vi "Field Setup.vi"(6 "path to png file":path=path "C:/Users/a0272913/Desktop/AppRawJSON/drawing.png", 10 "JSONCluster":T2, 11 "Zones In":T1[](array[typedef])) -> (2 "Field":picture, 3 "Zones Out":T1[](array[typedef]))   [LabVIEW 2015]
uses:
  Typedef/JSONCluster.ctl
  Typedef/Zone Data.ctl
panel:
  in  "Open Button":bool
  in  "Save Button":bool
  in  "Zones":i32(listbox)
  in  "Close":bool
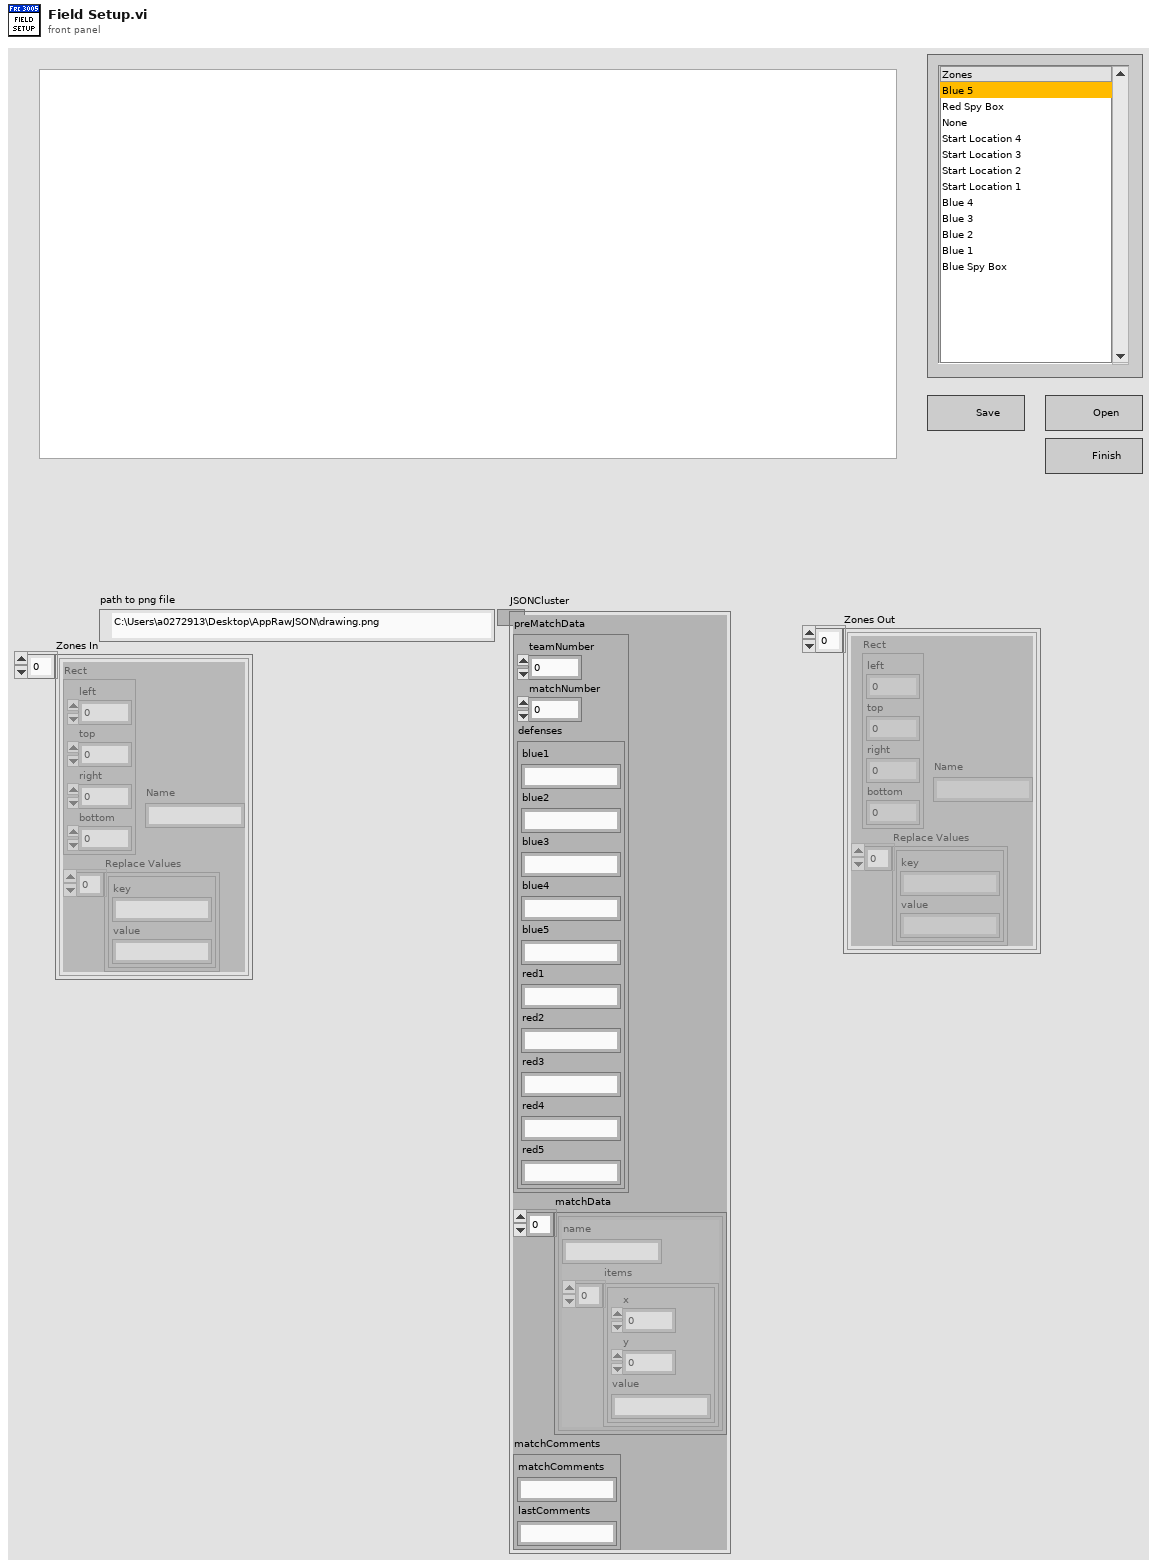
[diagram p1: front panel]
types:
  T1 = typedef "Zone Data.ctl" = cluster{"Rect":cluster{"left":i16, "top":i16, "right":i16, "bottom":i16}, "Replace Values":cluster{"key":string, "value":string}[], "Name":string}
  T2 = typedef "JSONCluster.ctl" = cluster{"preMatchData":cluster{"teamNumber":i32, "matchNumber":i32, "defenses":cluster{"blue1":string, "blue2":string, "blue3":string, "blue4":string, "blue5":string, "red1":string, "red2":string, "red3":string, "red4":string, "red5":string}}, "matchData":cluster{"name":string, "items":cluster{"x":i32, "y":i32, "value":string}[]}[], "matchComments":cluster{"matchComments":string, "lastComments":string}}
  T3 = cluster{"Field":picture, "Zone Active?":bool, "StoredField":picture, "Active Zone":cluster{"TLx":i16, "TLy":i16, "BRx":i16, "BRy":i16}, "Zones":T1[]}
  T4 = typedef "LVBoundsTypeDef.ctl" = cluster{"Width":u32, "Height":u32}
  T5 = typedef "imagedata.ctl" = cluster{"image type":i32, "image depth":i32, "image":u8[], "mask":u8[], "colors":u32[], "Rectangle":cluster{"left":i16, "top":i16, "right":i16, "bottom":i16}}
  T6 = cluster{"name":string, "items":cluster{"x":i32, "y":i32, "value":string}[]}[]
  T7 = typedef "LVMouseTypeDef.ctl" = cluster{"Mouse Position":cluster{"X":i32, "Y":i32}, "Mouse Modifiers":cluster{"Button Down":bool, "Shift Mod":bool, "Menu Mod":bool, "Option Mod":bool}}
  T8 = cluster{"TLx":i16, "TLy":i16, "BRx":i16, "BRy":i16}
  T9 = cluster{"left":i16, "top":i16, "right":i16, "bottom":i16}
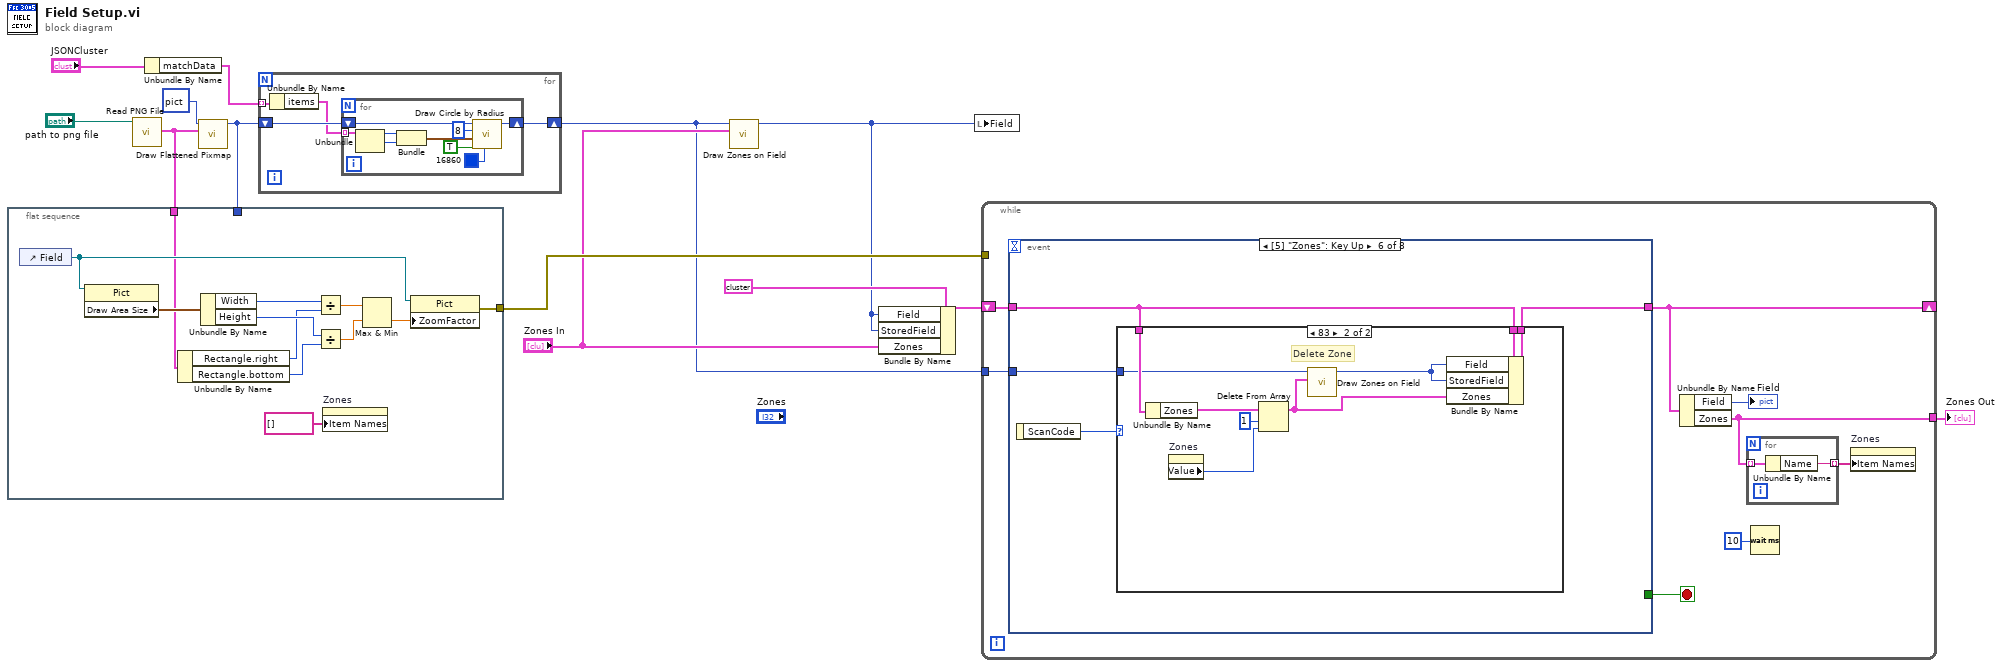
[diagram p0: block diagram]
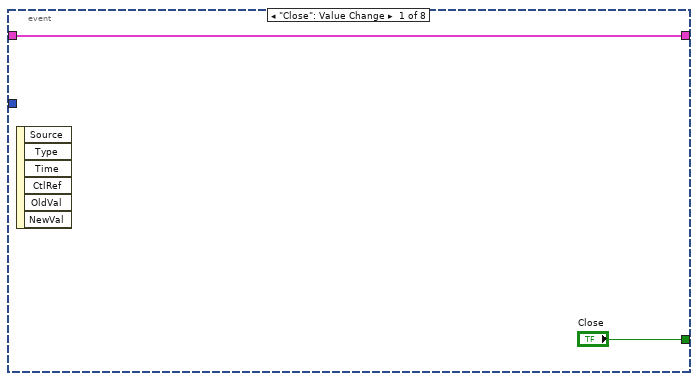
[diagram p2: hidden frame]
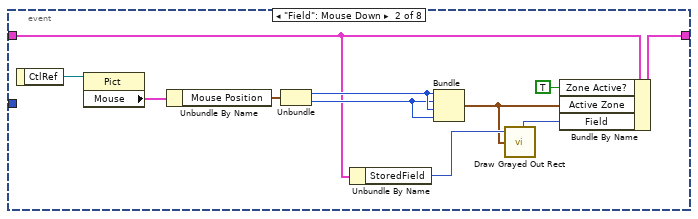
[diagram p3: hidden frame]
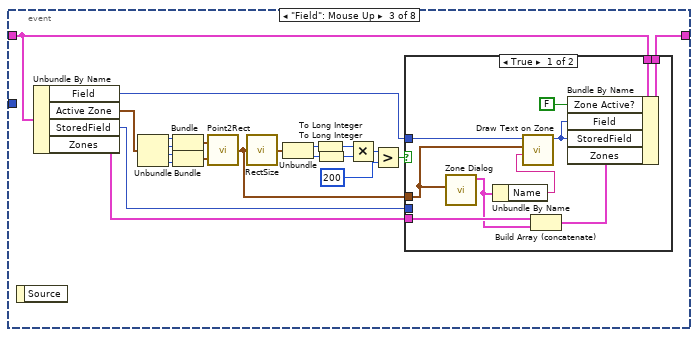
[diagram p4: hidden frame]
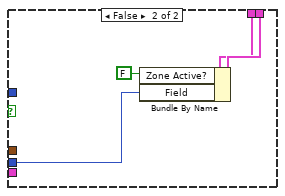
[diagram p5: hidden frame]
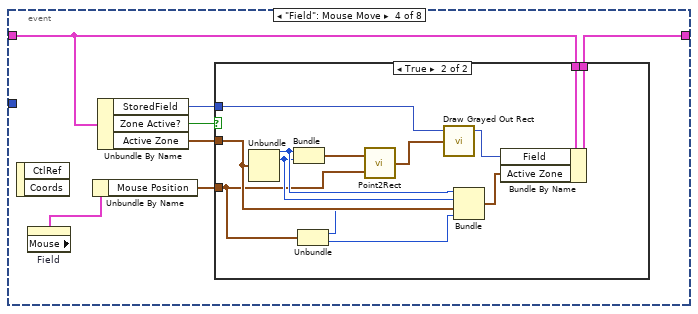
[diagram p6: hidden frame]
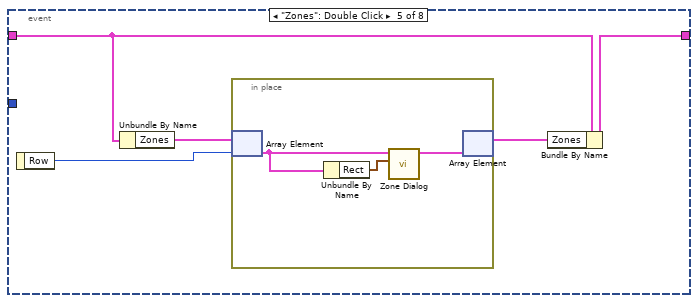
[diagram p8: hidden frame]
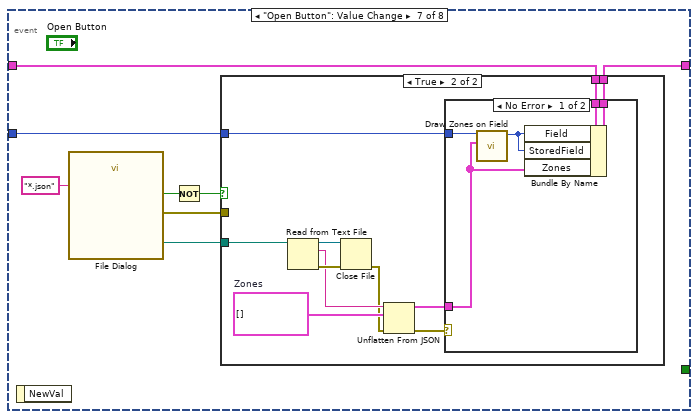
[diagram p10: hidden frame]
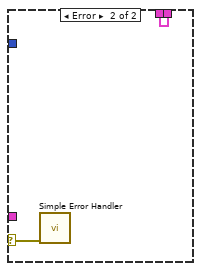
[diagram p12: hidden frame]
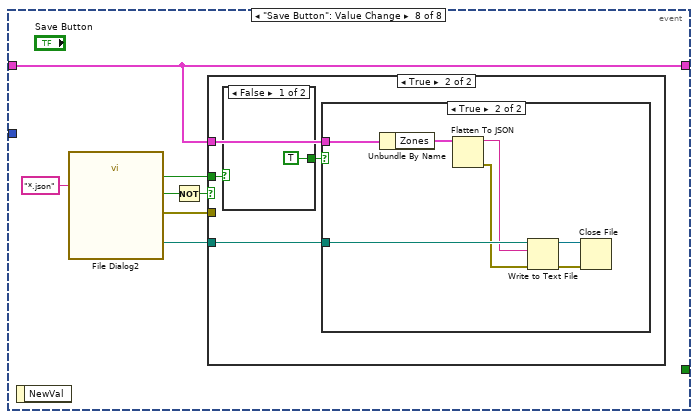
[diagram p13: hidden frame]
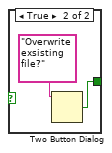
[diagram p15: hidden frame]
diagram:
  n1 = flat-sequence {
    tunnel: w12 -> [w16]
    tunnel: [w15] -> w7
    tunnel: w9 -> [_]
    frame #0 {
      n2 = control-ref of="Field"() -> (w17:refnum<vi>)
      n3 = property class="Pict"(reference=w17) -> ("Draw Area Size"=w22:T4)  [unwired: 1 in, 2 out]
      n4 = Unbundle By Name(w16) -> ("Rectangle.right"=w19:i16, "Rectangle.bottom"=w18:i16)
      n5 = Unbundle By Name(w22) -> ("Width"=w21:u32, "Height"=w20:u32)
      n6 = Divide(x=w21, y=w19) -> (x/y=w23:dbl)
      n7 = Divide(x=w20, y=w18) -> (x/y=w24:dbl)
      n8 = property on="Zones" class="LstBox (strict)"("Item Names"=string[] []) -> ()  [unwired: 2 in, 2 out]
      n9 = Max & Min(x=w23, y=w24) -> (min(x,y)=w25:dbl)  [unwired: 1 out]
      n10 = property class="Pict"(reference=w17, "ZoomFactor"=w25) -> (error out=w15:errorcluster)  [unwired: 1 in, 1 out]
    }
  }
  n11 = call <vilib>:"Read PNG File.vi"("path to PNG file"="path to png file") -> ("image data"=w12:T5)  [unwired: 8 in, 2 out]
  n12 = Unbundle By Name("JSONCluster") -> ("matchData"=w11:T6)
  n13 = call <vilib>:"Draw Flattened Pixmap.vi"("image data"=w12, "picture"=picture data[5B]) -> ("new picture"=w9:picture)  [unwired: 7 in]
  n14 = for {
    shift-right: [w28] -> w1
    shift-left: w9 -> [w29]
    tunnel: w11 -> [w27] mode=indexing
    n15 = Unbundle By Name(w27) -> ("items"=w26:cluster{"x":i32, "y":i32, "value":string}[])
    n16 = for {
      shift-right: [w37] -> w28
      shift-left: w29 -> [w38]
      tunnel: w26 -> [w33] mode=indexing
      n17 = Unbundle(w33) -> ("x"=w32:i32, "y"=w31:i32)  [unwired: 1 out]
      n18 = Bundle("x"=w32, "y"=w31) -> (w30:cluster{"x":i32, "y":i32})  [unwired: 1 in]
      n19 = call <vilib>:"Draw Circle by Radius.vi"("color(black)"=u32 16860, "fill?(F)"=TRUE, "pixel center"=w30, "radius"=i16 8, "picture"=w38) -> ("new picture"=w37:picture)  [unwired: 6 in]
    }
  }
  n20 = call "Draw Zones on Field.vi"("Zones In"="Zones In", "new picture in"=w1) -> ("new picture out"=w3:picture)  [unwired: 9 in]
  n21 = Bundle By Name(cluster=T3 {"Field"=bytes[0], "Zone Active?"=FALSE, "StoredField"=bytes[0], "Active Zone"={"TLx"=0, "TLy"=0, "BRx"=0, "BRy"=0}, "Zones"=[]}, "Field"=w3, "StoredField"=w3, "Zones"="Zones In") -> (w5:T3)
  n22 = local write "Field"(w3) -> ()
  n23 = while {
    tunnel: w7 -> [_]
    shift-right: [w45] -> _
    shift-left: w5 -> [w46]
    tunnel: [w40] -> w4
    tunnel: w1 -> [w39]
    stop <- w43 stop-if-true
    n24 = event shown="[5] \"Zones\": Key Up" {
      selector: _ -> [_ _ _ _ _ _ _ _]
      dyn-events: _ -> [_ _ _ _ _ _ _ _]
      timeout: _ -> [_ _ _ _ _ _ _ _]
      tunnel: w46 -> [w50 w58 w81 w101 w122 w127 w147 w169]
      tunnel: [w50 w61 w82 w100 w121 w128 w142 w169] -> w45
      tunnel: ["Close" _ _ _ _ _ _ _] -> w43
      tunnel: w39 -> [_ _ _ _ _ w126 w143 _]
      event "Close": Value Change {
        n25 = event-data() -> ()  [unwired: 1 in, 6 out]
      }
      event "Field": Mouse Down {
        n26 = event-data() -> ("CtlRef"=w53:refnum<vi>)  [unwired: 1 in]
        n27 = property on="Property Node" class="Pict"(reference=w53) -> ("Mouse"=w52:T7)  [unwired: 1 in, 2 out]
        n28 = Unbundle By Name(w52) -> ("Mouse Position"=w51:cluster{"X":i32, "Y":i32})
        n29 = Unbundle(w51) -> ("X"=w60:i32, "Y"=w59:i32)
        n30 = Unbundle By Name(w58) -> ("StoredField"=w57:picture)
        n31 = Bundle("X"=w60, "Y"=w59, "X"=w60, "Y"=w59) -> (w55:cluster{"X":i32, "Y":i32, "X":i32, "Y":i32})  [unwired: 1 in]
        n32 = call <vilib>:"Draw Grayed Out Rect.vi"("rect"=w55, "picture"=w57) -> ("new picture"=w56:picture)  [unwired: 3 in]
        n33 = Bundle By Name(cluster=w58, "Zone Active?"=TRUE, "Active Zone"=w55, "Field"=w56) -> (w61:T3)
      }
      event "Field": Mouse Up {
        n34 = event-data() -> ()  [unwired: 1 in, 1 out]
        n35 = Unbundle By Name(w81) -> ("Field"=w80:picture, "Active Zone"=w79:T8, "StoredField"=w66:picture, "Zones"=w63:T1[])
        n36 = Unbundle(w79) -> ("TLx"=w78:i16, "TLy"=w77:i16, "BRx"=w76:i16, "BRy"=w75:i16)
        n37 = Bundle("TLx"=w78, "TLy"=w77) -> (w74:cluster{"TLx":i16, "TLy":i16})  [unwired: 1 in]
        n38 = Bundle("BRx"=w76, "BRy"=w75) -> (w73:cluster{"BRx":i16, "BRy":i16})  [unwired: 1 in]
        n39 = call <vilib>:"Point2Rect.vi"("point b"=w73, "point a"=w74) -> ("rect"=w62:T9)
        n40 = call <vilib>:"RectSize.vi"("rect"=w62) -> ("point"=w72:cluster{"x":i16, "y":i16})
        n41 = Unbundle(w72) -> ("x"=w70:i16, "y"=w71:i16)
        n42 = To Long Integer(number=w70) -> (32bit integer=w65:i32)
        n43 = To Long Integer(number=w71) -> (32bit integer=w64:i32)
        n44 = Multiply(x=w65, y=w64) -> (x*y=w69:i32)
        n45 = Greater?(x=w69, y=200) -> (0:w67:bool)
        n46 = case shown="True" w67 {
          tunnel: [w92 w96] -> w82
          tunnel: w81 -> [w91 w94]
          tunnel: w80 -> [w88 _]
          tunnel: w66 -> [_ w93]
          tunnel: w63 -> [w90 _]
          tunnel: w62 -> [w85 _]
          frame True {
            n47 = call "Zone Dialog.vi"("Rect"=w85) -> ("Zone"=w87:T1)  [unwired: 10 in]
            n48 = Unbundle By Name(w87) -> ("Name"=w86:string)
            n49 = call "Draw Text on Zone.vi"("Name"=w86, "rect"=w85, "Field"=w88) -> ("new picture"=w83:picture)  [unwired: 8 in]
            n50 = Build Array (concatenate)(w90, w87) -> (w89:T1[])
            n51 = Bundle By Name(cluster=w91, "Zone Active?"=FALSE, "Field"=w83, "StoredField"=w83, "Zones"=w89) -> (w92:T3)
          }
          frame False {
            n52 = Bundle By Name(cluster=w94, "Zone Active?"=FALSE, "Field"=w93) -> (w96:T3)
          }
        }
      }
      event "Field": Mouse Move {
        n53 = event-data() -> ()  [unwired: 1 in, 2 out]
        n54 = property on="Field" class="Pict"() -> ("Mouse"=w98:T7)  [unwired: 2 in, 2 out]
        n55 = Unbundle By Name(w98) -> ("Mouse Position"=w97:cluster{"X":i32, "Y":i32})
        n56 = Unbundle By Name(w101) -> ("StoredField"=w99:picture, "Zone Active?"=w103:bool, "Active Zone"=w102:T8)
        n57 = case shown="True" w103 {
          tunnel: w102 -> [_ w111]
          tunnel: w97 -> [_ w108]
          tunnel: w101 -> [w104 w116]
          tunnel: [w104 w115] -> w100
          tunnel: w99 -> [_ w114]
          frame False {
          }
          frame True {
            n58 = Unbundle(w111) -> ("TLx"=w110:i16, "TLy"=w109:i16)  [unwired: 2 out]
            n59 = Bundle("TLx"=w110, "TLy"=w109) -> (w117:cluster{"TLx":i16, "TLy":i16})  [unwired: 1 in]
            n60 = Unbundle(w108) -> ("X"=w107:i32, "Y"=w106:i32)
            n61 = call <vilib>:"Point2Rect.vi"("point b"=w108, "point a"=w117) -> ("rect"=w112:T9)
            n62 = call <vilib>:"Draw Grayed Out Rect.vi"("rect"=w112, "picture"=w114) -> ("new picture"=w113:picture)  [unwired: 3 in]
            n63 = Bundle(cluster=w111, "TLx"=w110, "TLy"=w109, "BRx"=w107, "BRy"=w106) -> (w105:T8)
            n64 = Bundle By Name(cluster=w116, "Field"=w113, "Active Zone"=w105) -> (w115:T3)
          }
        }
      }
      event "Zones": Double Click {
        n65 = event-data() -> ("Row"=w119:i32)  [unwired: 1 in]
        n66 = Unbundle By Name(w122) -> ("Zones"=w120:T1[])
        n67 = in-place {
          n68 = in-place-array #1(w120, w119) -> (w124:T1)
          n69 = Unbundle By Name(w124) -> ("Rect"=w125:T9)
          n70 = call "Zone Dialog.vi"("Rect"=w125, "Zone in"=w124) -> ("Zone"=w123:T1)  [unwired: 9 in]
          n71 = in-place-array #1(w123) -> (w118:T1[])  [unwired: 1 out]
        }
        n72 = Bundle By Name(cluster=w122, "Zones"=w118) -> (w121:T3)
      }
      event "Zones": Key Up {
        n73 = event-data() -> ("ScanCode"=w129:i16)  [unwired: 1 in]
        n74 = case shown="83" w129 {
          tunnel: w127 -> [w130 w138]
          tunnel: [w130 w139] -> w128
          tunnel: w127 -> [_ w137]
          tunnel: w126 -> [_ w136]
          frame 0, Default {
          }
          frame 83 {
            # "Delete Zone"
            n75 = Unbundle By Name(w137) -> ("Zones"=w135:T1[])
            n76 = property on="Zones" class="LstBox (strict)"() -> ("Value"=w133:i32)  [unwired: 2 in, 2 out]
            n77 = Delete From Array(array=w135, length=1, index=w133) -> (array with subset deleted=w131:T1[])  [unwired: 1 out]
            n78 = call "Draw Zones on Field.vi"("Zones In"=w131, "new picture in"=w136) -> ("new picture out"=w134:picture)  [unwired: 9 in]
            n79 = Bundle By Name(cluster=w138, "Field"=w134, "StoredField"=w134, "Zones"=w131) -> (w139:T3)
          }
        }
      }
      event "Open Button": Value Change {
        n80 = event-data() -> ()  [unwired: 1 in, 1 out]
        n81 = call "File Dialog"("pattern (all files)"="*.json") -> ("selected path"=w145:path, "cancelled"=w144:bool, "error out"=w140:errorcluster)  [unwired: 11 in, 1 out]
        n82 = Not(x=w144) -> (.not. x?=w141:bool)
        n83 = case shown="True" w141 {
          tunnel: w147 -> [w148 w159]
          tunnel: w145 -> [_ w158]
          tunnel: w143 -> [_ w157]
          tunnel: [w148 w156] -> w142
          tunnel: w140 -> [_ _]
          frame False {
          }
          frame True {
            w154 = T1[] []  # Zones
            n84 = Read from Text File(file (use dialog)=w158) -> (refnum out=w152:refnum<file>, text=w151:string, error out=w153:errorcluster)  [unwired: 3 in, 1 out]
            n85 = Close File(refnum=w152, error in=w153) -> (error out=w150:errorcluster)  [unwired: 1 out]
            n86 = Unflatten From JSON(JSON string=w151, type and defaults=w154, error in (no error)=w150) -> (value=w155:T1[], error out=w149:errorcluster)  [unwired: 4 in]
            n87 = case shown="No Error" w149 {
              selector: w149 -> [_ w165]
              tunnel: w159 -> [w164 w166]
              tunnel: w157 -> [w163 _]
              tunnel: [w162 w166] -> w156
              tunnel: w155 -> [w160 _]
              frame No Error {
                n88 = call "Draw Zones on Field.vi"("Zones In"=w160, "new picture in"=w163) -> ("new picture out"=w161:picture)  [unwired: 9 in]
                n89 = Bundle By Name(cluster=w164, "Field"=w161, "StoredField"=w161, "Zones"=w160) -> (w162:T3)
              }
              frame Error {
                n90 = call <vilib>:"Simple Error Handler.vi"("error in (no error)"=w165) -> ()  [unwired: 4 in, 5 out]
              }
            }
          }
        }
      }
      event "Save Button": Value Change {
        n91 = event-data() -> ()  [unwired: 1 in, 1 out]
        n92 = call "File Dialog2"("pattern (all files)"="*.json") -> ("selected path"=w172:path, "exists"=w167:bool, "cancelled"=w171:bool, "error out"=w168:errorcluster)  [unwired: 11 in]
        n93 = Not(x=w171) -> (.not. x?=w170:bool)
        n94 = case shown="True" w170 {
          tunnel: w172 -> [_ w177]
          tunnel: w169 -> [_ w176]
          tunnel: w168 -> [_ _]
          tunnel: w167 -> [_ w174]
          frame False {
          }
          frame True {
            n95 = case shown="False" w174 {
              tunnel: [TRUE ("T button?") w179] -> w175
              frame False {
              }
              frame True {
                n96 = Two Button Dialog(message="Overwrite exsisting file?") -> (T button?=w179:bool)  [unwired: 2 in]
              }
            }
            n97 = case shown="True" w175 {
              tunnel: w177 -> [_ w187]
              tunnel: w176 -> [_ w184]
              frame False {
              }
              frame True {
                n98 = Unbundle By Name(w184) -> ("Zones"=w183:T1[])
                n99 = Flatten To JSON(anything=w183) -> (JSON string=w182:string, 11:w181:errorcluster)  [unwired: 2 in]
                n100 = Write to Text File(file (use dialog)=w187, text=w182, error in=w181) -> (refnum out=w185:refnum<file>, error out=w186:errorcluster)  [unwired: 1 in, 1 out]
                n101 = Close File(refnum=w185, error in=w186) -> ()  [unwired: 2 out]
              }
            }
          }
        }
      }
    }
    n102 = Unbundle By Name(w45) -> ("Field"=→"Field":picture, "Zones"=w40:T1[])
    n103 = for {
      tunnel: w40 -> [w48] mode=indexing
      tunnel: [w47] -> w41 mode=indexing
      n104 = Unbundle By Name(w48) -> ("Name"=w47:string)
    }
    n105 = Wait (ms)(milliseconds to wait=u32 10) -> ()  [unwired: 1 out]
    n106 = property on="Zones" class="LstBox (strict)"("Item Names"=w41) -> ()  [unwired: 2 in, 2 out]
  }
  "Zones Out" <- w4
